vi "Get_Auth_URL.vi"(8 "error in (no error)":errorcluster, 11 "Asana in":refnum<class "Asana.lvclass">) -> (0 "error out":errorcluster, 3 "Asana out":refnum<class "Asana.lvclass">)   [LabVIEW 2016, in "Asana.lvclass"]
uses:
  Asana.lvclass
  Asana.lvclass/Asana.ctl
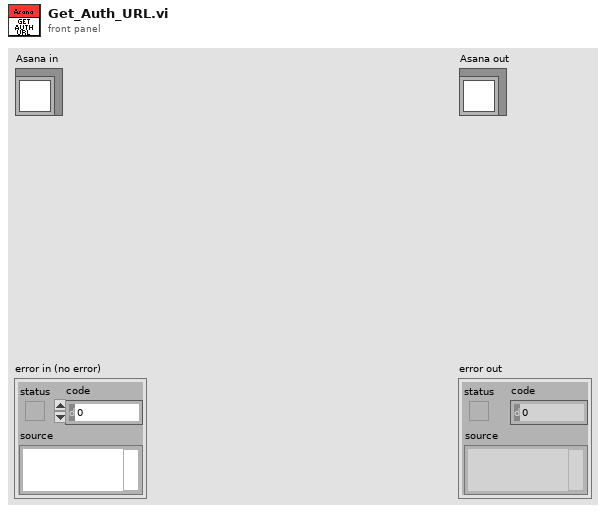
[diagram p1: front panel]
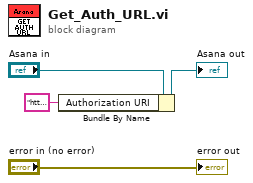
[diagram p0: block diagram]
diagram:
  n1 = Bundle By Name(cluster="Asana in", "Authorization URI"="https://app.asana.com/-/oauth_authorize?response_type=code&client_id=1108428692000476&redirect_uri=https%3A%2F%2Fapp.asana.com%2Fapi%2F1.0") -> (→"Asana out":refnum<class "Asana.lvclass">)
  "error out" <- "error in (no error)"
